vi "motor control.vi"(8 "speed":dbl, 11 "Reverse":bool) -> (2 "Voltage":dbl)   [LabVIEW 2017]
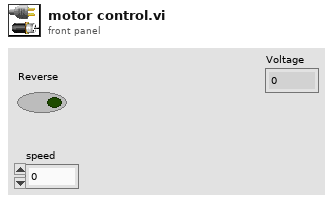
[diagram p1: front panel]
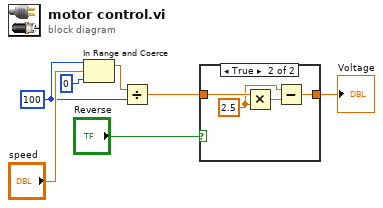
[diagram p0: block diagram]
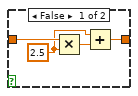
[diagram p2: hidden frame]
diagram:
  w2 = 100
  n1 = In Range and Coerce(upper limit=w2, x="speed", lower limit=0) -> (coerced(x)=w4:dbl)  [unwired: 1 out]
  n2 = Divide(x=w4, y=w2) -> (x/y=w5:dbl)
  n3 = case shown="True" "Reverse" {
    tunnel: w5 -> [w11 w14]
    tunnel: [w9 w13] -> w6
    frame False {
      w8 = 2.5
      n4 = Multiply(x=w11, y=w8) -> (x*y=w10:dbl)
      n5 = Add(x=w8, y=w10) -> (x+y=w9:dbl)
    }
    frame True {
      w12 = 2.5
      n6 = Multiply(x=w14, y=w12) -> (x*y=w15:dbl)
      n7 = Subtract(x=w12, y=w15) -> (x-y=w13:dbl)
    }
  }
  "Voltage" <- w6
